vi "Steppers_and_Scanners_control_6_14.vi"(1 "ANC300 address":refnum<visa-resource-name>="COM8") -> (18 "Serial":string="ANC300B-C-2133-4009033")   [LabVIEW 2023]
panel:
  in  "wait time (ms)":u32=50
  out "2: Voltage Reading":dbl format="%#_13g"
  out "1: Voltage Reading":dbl format="%#_13g"
  in  "Set/Read":bool
  in  "Stepper 4":bool
  in  "4: ms to wait":u32=1
  in  "4: number of steps":i32=1
  in  "4: stepping direction":bool=TRUE
  in  "4: AC Voltage":dbl=30.0 min=0.0 format="%.1g"
  in  "4: AC frequency":dbl=350.0 min=0.0 format="%.1f"
  in  "Stepper 3":bool
  in  "3: ms to wait":u32=1
  in  "3: number of steps":i32=1
  in  "3: stepping direction":bool=TRUE
  in  "3: AC Voltage":dbl=30.0 min=0.0 format="%.1g"
  in  "3: AC frequency":dbl=350.0 min=0.0 format="%.1f"
  in  "2: ms to wait":u32=50
  in  "2: Offset Voltage":dbl min=0.0 format="%.1g"
  in  "1: ms to wait":u32=50
  in  "1: Offset Voltage":dbl min=0.0 format="%.1g"
  # "Scanner 1"
  # "Scanner 2"
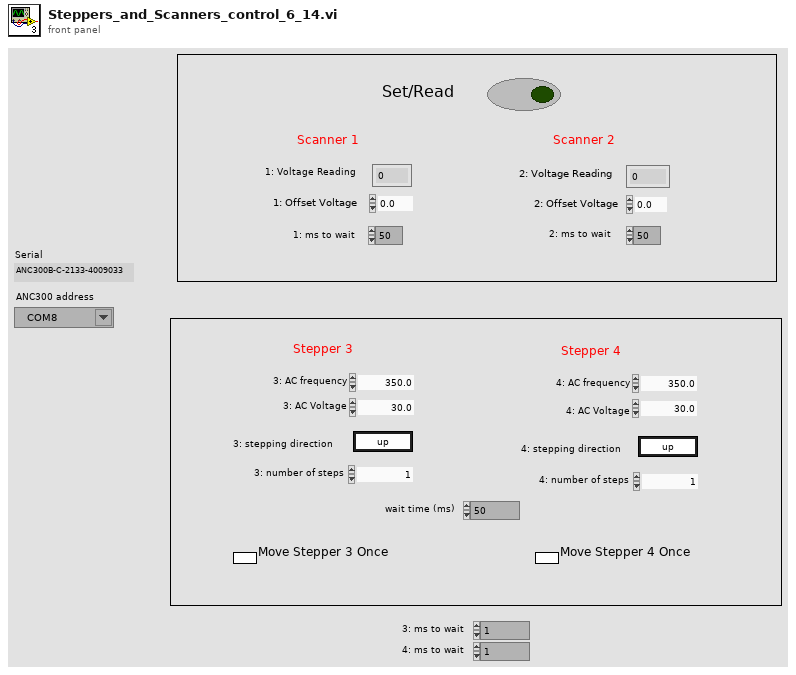
[diagram p1: front panel]
types:
  T1 = cluster{"error ":bool, "error number":i32, "error code":string}
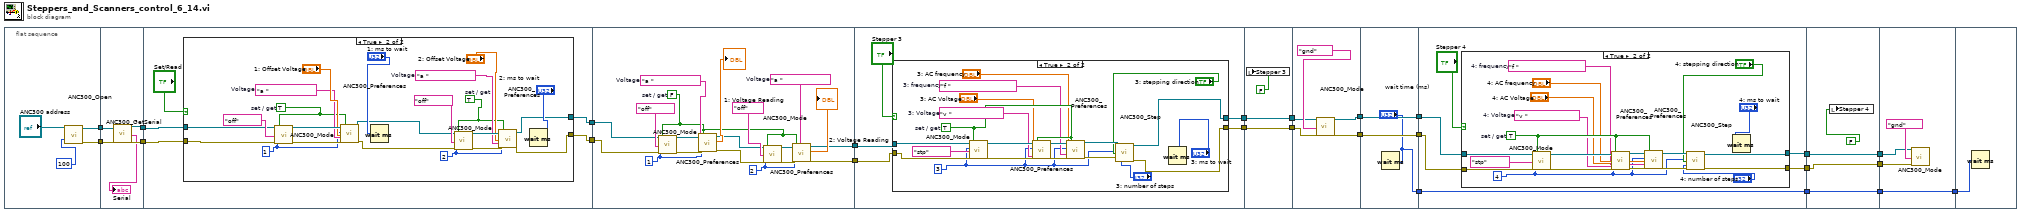
[diagram p0: block diagram]
diagram:
  n1 = flat-sequence {
    tunnel: [w26] -> w24
    tunnel: [w25] -> w23
    tunnel: [w32] -> w22
    tunnel: w24 -> [w33]
    tunnel: [w31] -> w21
    tunnel: w23 -> [w30]
    tunnel: [w38] -> w20
    tunnel: [w37] -> w19
    tunnel: w22 -> [w34]
    tunnel: w21 -> [w35]
    tunnel: w20 -> [w66]
    tunnel: w19 -> [w71]
    tunnel: [w64] -> w18
    tunnel: [w63] -> w17
    tunnel: w18 -> [w83]
    tunnel: w17 -> [w82]
    tunnel: [w85] -> w16
    tunnel: [w84] -> w15
    tunnel: w16 -> [w109]
    tunnel: w15 -> [w110]
    tunnel: [w110] -> w14
    tunnel: [w109] -> w13
    tunnel: w14 -> [w115]
    tunnel: w13 -> [w113]
    tunnel: [w114] -> w12
    tunnel: [w112] -> w11
    tunnel: w12 -> [w119]
    tunnel: w11 -> [w118]
    tunnel: [w119] -> w10
    tunnel: [w118] -> w9
    tunnel: ["wait time (ms)"] -> w8
    tunnel: w10 -> [w123]
    tunnel: w9 -> [w124]
    tunnel: [w122] -> w7
    tunnel: [w121] -> w6
    tunnel: w8 -> [w120]
    tunnel: [w120] -> w5
    tunnel: w7 -> [w150]
    tunnel: w6 -> [w149]
    tunnel: [w150] -> w4
    tunnel: [w149] -> w3
    tunnel: w5 -> [w148]
    tunnel: [w148] -> w2
    tunnel: w4 -> [w154]
    tunnel: w3 -> [w153]
    tunnel: w2 -> [w152]
    tunnel: [w152] -> w1
    tunnel: w1 -> [w156]
    frame #0 {
      n2 = call "ANC300_Open.vi"("ANC300 Communication Port In"="ANC300 address", "milliseconds to wait"=u32 100 ("millisecond timer value")) -> ("ANC300 Communication Port Out"=w26:refnum<visa-resource-name>, "error out"=w25:T1)  [unwired: 13 in, 3 out]
    }
    frame #1 {
      n3 = call "ANC300_GetSerial.vi"("ANC300 Communication Port In"=w33, "error in"=w30) -> ("ANC300 Communication Port Out"=w32:refnum<visa-resource-name>, "Serial"=→"Serial":string, "error out"=w31:T1)  [unwired: 10 in, 5 out]
    }
    frame #2 {
      n4 = case shown="True" "Set/Read" {
        tunnel: w35 -> [w39 w45]
        tunnel: w34 -> [w40 w46]
        tunnel: [w40 w41] -> w38
        tunnel: [w39 w42] -> w37
        frame False {
        }
        frame True {
          w47 = 2
          w48 = 1
          w49 = TRUE  # set / get
          w52 = "a "  # Voltage
          w56 = TRUE  # set / get
          w59 = "a "  # Voltage
          n5 = call "ANC300_Mode.vi"("ANC300 Communication Port In"=w46, "Axis"=w48, "axis mode in"="off", "error in"=w45, "set / get"=w56) -> ("ANC300 Communication Port Out"=w62:refnum<visa-resource-name>, "error out"=w61:T1)  [unwired: 8 in, 5 out]
          n6 = call "ANC300_Preferences.vi"("ANC300 Communication Port In"=w62, "Axis"=w48, "value in"="1: Offset Voltage", "parameter"=w59, "error in"=w61, "set / get"=w56) -> ("ANC300 Communication Port Out"=w44:refnum<visa-resource-name>, "error out"=w43:T1)  [unwired: 6 in, 6 out]
          n7 = Wait (ms)(milliseconds to wait="1: ms to wait") -> ()  [unwired: 1 out]
          n8 = call "ANC300_Mode.vi"("ANC300 Communication Port In"=w44, "Axis"=w47, "axis mode in"="off", "error in"=w43, "set / get"=w49) -> ("ANC300 Communication Port Out"=w55:refnum<visa-resource-name>, "error out"=w54:T1)  [unwired: 8 in, 5 out]
          n9 = call "ANC300_Preferences.vi"("ANC300 Communication Port In"=w55, "Axis"=w47, "value in"="2: Offset Voltage", "parameter"=w52, "error in"=w54, "set / get"=w49) -> ("ANC300 Communication Port Out"=w41:refnum<visa-resource-name>, "error out"=w42:T1)  [unwired: 6 in, 6 out]
          n10 = Wait (ms)(milliseconds to wait="2: ms to wait") -> ()  [unwired: 1 out]
        }
      }
    }
    frame #3 {
      w72 = 2
      w73 = 1
      w75 = "a "  # Voltage
      w68 = FALSE  # set / get
      w79 = "a "  # Voltage
      n11 = call "ANC300_Mode.vi"("ANC300 Communication Port In"=w66, "Axis"=w73, "axis mode in"="off", "error in"=w71, "set / get"=w68) -> ("ANC300 Communication Port Out"=w81:refnum<visa-resource-name>, "error out"=w80:T1)  [unwired: 8 in, 5 out]
      n12 = call "ANC300_Preferences.vi"("ANC300 Communication Port In"=w81, "Axis"=w73, "parameter"=w79, "error in"=w80, "set / get"=w68) -> ("ANC300 Communication Port Out"=w65:refnum<visa-resource-name>, "value out"=→"1: Voltage Reading":dbl, "error out"=w67:T1)  [unwired: 7 in, 5 out]
      n13 = call "ANC300_Mode.vi"("ANC300 Communication Port In"=w65, "Axis"=w72, "axis mode in"="off", "error in"=w67, "set / get"=w68) -> ("ANC300 Communication Port Out"=w77:refnum<visa-resource-name>, "error out"=w76:T1)  [unwired: 8 in, 5 out]
      n14 = call "ANC300_Preferences.vi"("ANC300 Communication Port In"=w77, "Axis"=w72, "parameter"=w75, "error in"=w76, "set / get"=w68) -> ("ANC300 Communication Port Out"=w64:refnum<visa-resource-name>, "value out"=→"2: Voltage Reading":dbl, "error out"=w63:T1)  [unwired: 7 in, 5 out]
    }
    frame #4 {
      n15 = case shown="True" "Stepper 3" {
        tunnel: w83 -> [w88 w108]
        tunnel: [w88 w90] -> w85
        tunnel: [w87 w92] -> w84
        tunnel: w82 -> [w87 w91]
        frame False {
        }
        frame True {
          w89 = 3
          w94 = "v "  # 3: Voltage
          w96 = "f "  # 3: frequency
          w99 = TRUE  # set / get
          n16 = call "ANC300_Mode.vi"("ANC300 Communication Port In"=w108, "Axis"=w89, "axis mode in"="stp", "error in"=w91, "set / get"=w99) -> ("ANC300 Communication Port Out"=w107:refnum<visa-resource-name>, "error out"=w105:T1)  [unwired: 8 in, 5 out]
          n17 = call "ANC300_Preferences.vi"("ANC300 Communication Port In"=w107, "Axis"=w89, "value in"="3: AC Voltage", "parameter"=w94, "error in"=w105, "set / get"=w99) -> ("ANC300 Communication Port Out"=w103:refnum<visa-resource-name>, "error out"=w102:T1)  [unwired: 6 in, 6 out]
          n18 = call "ANC300_Preferences.vi"("ANC300 Communication Port In"=w103, "Axis"=w89, "value in"="3: AC frequency", "parameter"=w96, "error in"=w102, "set / get"=w99) -> ("ANC300 Communication Port Out"=w106:refnum<visa-resource-name>, "error out"=w104:T1)  [unwired: 6 in, 6 out]
          n19 = call "ANC300_Step.vi"("ANC300 Communication Port In"=w106, "Axis"=w89, "stepping direction"="3: stepping direction", "number of steps [0=cont.]"="3: number of steps", "error in"=w104) -> ("ANC300 Communication Port Out"=w90:refnum<visa-resource-name>, "error out"=w92:T1)  [unwired: 9 in, 4 out]
          n20 = Wait (ms)(milliseconds to wait="3: ms to wait") -> ()  [unwired: 1 out]
        }
      }
    }
    frame #5 {
      n21 = local write "Stepper 3"(FALSE) -> ()
    }
    frame #6 {
      n22 = call "ANC300_Mode.vi"("ANC300 Communication Port In"=w113, "axis mode in"="gnd" ("3 Stepper x"), "error in"=w115) -> ("ANC300 Communication Port Out"=w112:refnum<visa-resource-name>, "error out"=w114:T1)  [unwired: 10 in, 5 out]
    }
    frame #7 {
      n23 = Wait (ms)(milliseconds to wait="wait time (ms)") -> ()  [unwired: 1 out]
    }
    frame #8 {
      n24 = case shown="True" "Stepper 4" {
        tunnel: w124 -> [w127 w147]
        tunnel: w123 -> [w126 w144]
        tunnel: [w127 w139] -> w122
        tunnel: [w126 w129] -> w121
        frame False {
        }
        frame True {
          w128 = 4
          w134 = "v "  # 4: Voltage
          w132 = "f "  # 4: frequency
          w136 = TRUE  # set / get
          n25 = call "ANC300_Mode.vi"("ANC300 Communication Port In"=w147, "Axis"=w128, "axis mode in"="stp", "error in"=w144, "set / get"=w136) -> ("ANC300 Communication Port Out"=w146:refnum<visa-resource-name>, "error out"=w143:T1)  [unwired: 8 in, 5 out]
          n26 = call "ANC300_Preferences.vi"("ANC300 Communication Port In"=w146, "Axis"=w128, "value in"="4: AC Voltage", "parameter"=w134, "error in"=w143, "set / get"=w136) -> ("ANC300 Communication Port Out"=w141:refnum<visa-resource-name>, "error out"=w140:T1)  [unwired: 6 in, 6 out]
          n27 = call "ANC300_Preferences.vi"("ANC300 Communication Port In"=w141, "Axis"=w128, "value in"="4: AC frequency", "parameter"=w132, "error in"=w140, "set / get"=w136) -> ("ANC300 Communication Port Out"=w145:refnum<visa-resource-name>, "error out"=w142:T1)  [unwired: 6 in, 6 out]
          n28 = call "ANC300_Step.vi"("ANC300 Communication Port In"=w145, "Axis"=w128, "stepping direction"="4: stepping direction", "number of steps [0=cont.]"="4: number of steps", "error in"=w142) -> ("ANC300 Communication Port Out"=w139:refnum<visa-resource-name>, "error out"=w129:T1)  [unwired: 9 in, 4 out]
          n29 = Wait (ms)(milliseconds to wait="4: ms to wait") -> ()  [unwired: 1 out]
        }
      }
    }
    frame #9 {
      n30 = local write "Stepper 4"(FALSE) -> ()
    }
    frame #10 {
      n31 = call "ANC300_Mode.vi"("ANC300 Communication Port In"=w154, "axis mode in"="gnd" ("3 Stepper x"), "error in"=w153) -> ()  [unwired: 10 in, 7 out]
    }
    frame #11 {
      n32 = Wait (ms)(milliseconds to wait=w156) -> ()  [unwired: 1 out]
    }
  }
